vi "Fake Test.vi"() -> ()   [LabVIEW 2017, in "LVUnit Test Executor.Tests.lvlib"]
uses:
  LVUnit Test Executor.Tests.lvlib
panel:
  out "error out":errorcluster
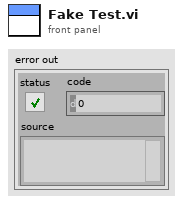
[diagram p1: front panel]
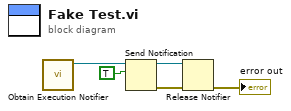
[diagram p0: block diagram]
diagram:
  n1 = call "Obtain Execution Notifier.vi"() -> ("Execution Notifier"=w5:refnum<notifier>)  [unwired: 11 in]
  n2 = Send Notification(notification=TRUE, notifier=w5) -> (notifier out=w3:refnum<notifier>, error out=w2:errorcluster)  [unwired: 1 in]
  n3 = Release Notifier(notifier=w3, error in (no error)=w2) -> (error out=→"error out":errorcluster)  [unwired: 1 in, 2 out]
